vi "gen_stack_func.vi"(8 "error in (no error)":errorcluster, 11 "TrajectoryAK101022Resonance in":refnum<class "TrajectoryAK101022Resonance.lvclass">) -> (0 "error out":errorcluster, 2 "z-Points Array":dbl[unit][](array[numeric]), 3 "TrajectoryAK101022Resonance out":refnum<class "TrajectoryAK101022Resonance.lvclass">)   [LabVIEW 2010, in "TrajectoryAK101022Resonance.lvclass"]
uses:
  TrajectoryAK101022Resonance.lvclass
  TrajectoryAK101022Resonance.lvclass/TrajectoryAK101022Resonance.ctl
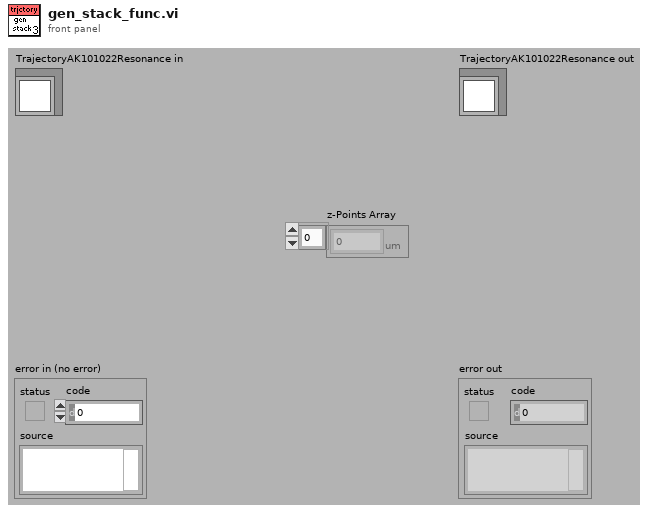
[diagram p1: front panel]
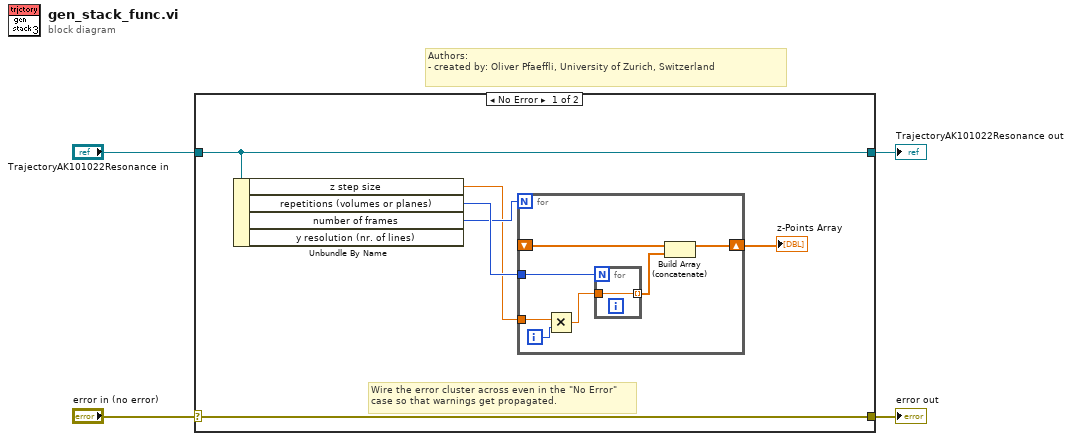
[diagram p0: block diagram]
diagram:
  # "Authors: \n- created by: Oliver Pfaeffli, University of Zurich, Switzerland"
  n1 = case shown="No Error" "error in (no error)" {
    selector: "error in (no error)" -> [w10 w20]
    tunnel: [w10 w20] -> w3
    tunnel: [w9 w19] -> w1
    tunnel: "TrajectoryAK101022Resonance in" -> [w9 w19]
    frame No Error {
      # "Wire the error cluster across even in the \"No Error\"\ncase so that warnings get propagated."
      n2 = Unbundle By Name(w9) -> ("z step size"=w6:dbl[unit], "repetitions (volumes or planes)"=w8:i32, "number of frames"=w7:i32)  [unwired: 1 out]
      n3 = for {
        N: w7 -> [_]
        tunnel: w8 -> [w17]
        tunnel: w6 -> [w15]
        shift-right: [w12] -> w5
        shift-left: _ -> [w11]
        i -> [w16]
        n4 = Multiply(x=w15, y=w16) -> (x*y=w14:dbl[unit])
        n5 = for {
          N: w17 -> [_]
          tunnel: w14 -> [w18]
          tunnel: [w18] -> w13 mode=indexing
        }
        n6 = Build Array (concatenate)(w11, w13) -> (w12:dbl[unit][])
      }
      "z-Points Array" <- w5
    }
    frame Error {
    }
  }
  "error out" <- w3
  "TrajectoryAK101022Resonance out" <- w1
